vi "Cursors2WindowCut.vi"(1 "Cursor List":T2) -> (0 "Window":T1)   [LabVIEW 2009]
uses:
  <vilib>/Utility/miscctls.llb/LVCursorListTypeDef.ctl
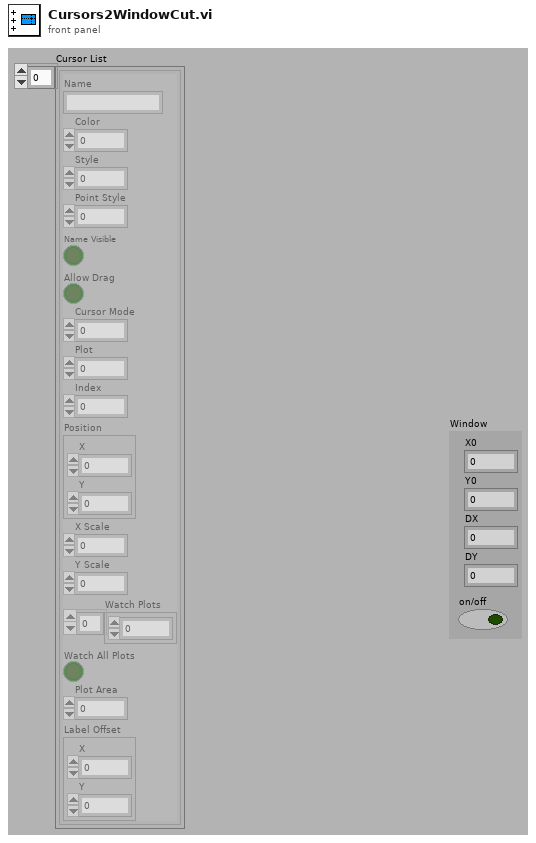
[diagram p1: front panel]
types:
  T1 = cluster{"X0":u16, "Y0":u16, "DX":u16, "DY":u16, "on/off":bool}
  T2 = typedef "LVCursorListTypeDef.ctl" = cluster{"Name":string, "Color":u32, "Style":u8, "Point Style":u8, "Name Visible":bool, "Allow Drag":bool, "Cursor Mode":u32, "Plot":i32, "Index":i32, "Position":cluster{"X":dbl, "Y":dbl}, "X Scale":u32, "Y Scale":u32, "Watch Plots":i32[], "Watch All Plots":bool, "Plot Area":i32, "Label Offset":cluster{"X":dbl, "Y":dbl}}[]
  T3 = cluster{"Name":string, "Color":u32, "Style":u8, "Point Style":u8, "Name Visible":bool, "Allow Drag":bool, "Cursor Mode":u32, "Plot":i32, "Index":i32, "Position":cluster{"X":dbl, "Y":dbl}, "X Scale":u32, "Y Scale":u32, "Watch Plots":i32[], "Watch All Plots":bool, "Plot Area":i32, "Label Offset":cluster{"X":dbl, "Y":dbl}}[]
  T4 = cluster{"Name":string, "Color":u32, "Style":u8, "Point Style":u8, "Name Visible":bool, "Allow Drag":bool, "Cursor Mode":u32, "Plot":i32, "Index":i32, "Position":cluster{"X":dbl, "Y":dbl}, "X Scale":u32, "Y Scale":u32, "Watch Plots":i32[], "Watch All Plots":bool, "Plot Area":i32, "Label Offset":cluster{"X":dbl, "Y":dbl}}
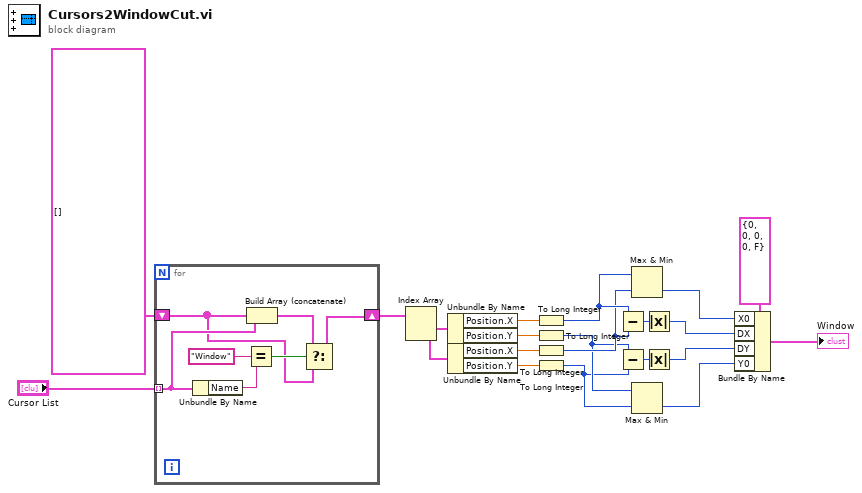
[diagram p0: block diagram]
diagram:
  n1 = for {
    tunnel: "Cursor List" -> [w25] mode=indexing
    shift-right: [w23] -> w1
    shift-left: T3 [] -> [w22]
    n2 = Unbundle By Name(w25) -> ("Name"=w28:string)
    n3 = Equal?(x="Window", y=w28) -> (x = y?=w26:bool)
    n4 = Build Array (concatenate)(w22, w25) -> (w24:T3)
    n5 = Select(t=w24, s=w26, f=w22) -> (s? t:f=w23:T3)
  }
  n6 = Index Array(array=w1) -> (element #1=w14:T4, element #2=w15:T4)  [unwired: 2 in]
  n7 = Unbundle By Name(w14) -> ("Position.X"=w16:dbl, "Position.Y"=w18:dbl)
  n8 = Unbundle By Name(w15) -> ("Position.X"=w17:dbl, "Position.Y"=w19:dbl)
  n9 = To Long Integer(number=w16) -> (32bit integer=w13:i32)
  n10 = To Long Integer(number=w18) -> (32bit integer=w11:i32)
  n11 = To Long Integer(number=w17) -> (32bit integer=w12:i32)
  n12 = To Long Integer(number=w19) -> (32bit integer=w10:i32)
  n13 = Subtract(x=w13, y=w12) -> (x-y=w20:i32)
  n14 = Subtract(x=w11, y=w10) -> (x-y=w21:i32)
  n15 = Max & Min(x=w13, y=w12) -> (min(x,y)=w7:i32)  [unwired: 1 out]
  n16 = Max & Min(x=w11, y=w10) -> (min(x,y)=w4:i32)  [unwired: 1 out]
  n17 = Absolute Value(x=w20) -> (abs(x)=w6:i32)
  n18 = Absolute Value(x=w21) -> (abs(x)=w5:i32)
  n19 = Bundle By Name(cluster=T1 {"X0"=0, "Y0"=0, "DX"=0, "DY"=0, "on/off"=FALSE} ("Window"), "X0"=w7, "DX"=w6, "DY"=w5, "Y0"=w4) -> (→"Window":T1)
